vi "Compile Directional Speed Settings.vi"(10 "Tooth centers":u16[](array[numeric]), 11 "APU start position":u16) -> (1 "upper index":fxp<+,10,10>, 2 "lower value":u16, 3 "upper value":u16, 4 "lower index":fxp<+,10,10>)   [LabVIEW 2019, in "Engine Simulation Toolkit System Explorer.lvlib"]
uses:
  Engine Simulation Toolkit System Explorer.lvlib
panel:
  # "60k should be\nupper value : 18k\nlower value : 54k\nupper idx : 0\nlower idx : 2"
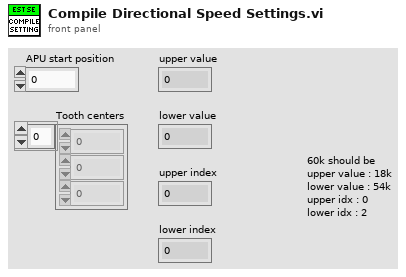
[diagram p1: front panel]
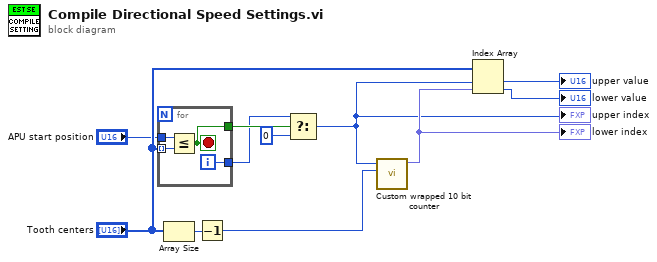
[diagram p0: block diagram]
diagram:
  n1 = for {
    tunnel: "APU start position" -> [w15]
    tunnel: "Tooth centers" -> [w14] mode=indexing
    tunnel: [w13] -> w3
    tunnel: [w12] -> w4
    i -> [w13]
    stop <- w12 stop-if-true
    n2 = Less Or Equal?(x=w15, y=w14) -> (x <= y?=w12:bool)
  }
  n3 = Array Size(array="Tooth centers") -> (size(s)=w6:i32)
  n4 = Decrement(x=w6) -> (x-1=w7:i32)
  n5 = Select(t=w3, s=w4, f=0) -> (s? t:f=w2:i32)
  "upper index" <- w2
  n6 = call "Custom wrapped 10 bit counter.vi"("max value"=w7, "value"=w2) -> ("new value"=w10:fxp<+,10,10>)  [unwired: 8 in, 1 out]
  "lower index" <- w10
  n7 = Index Array(array="Tooth centers", index #1=w2, index #2=w10) -> (element #1=→"upper value":u16, element #2=→"lower value":u16)
